vi "CaseStructure Create Case Calls.vi"(9 "Output variables assignements":string[](array[string]), 10 "Frames code[]":string[](array[string]), 11 "FrameNames in":string[](array[string])) -> (2 "Switch Cases C calls all as string":string, 3 "Switch Cases C string array":string[](array[string]))   [LabVIEW 2014]
doc: "Creates case calls for switch(){case \"someName\": break;} and returns them as array."
panel:
  # "Each case \"\" has output variables, so there is way how to get some value from them."
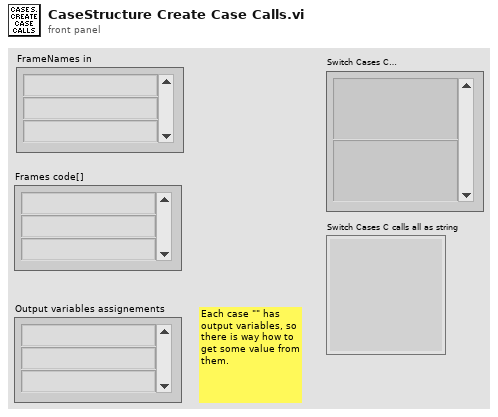
[diagram p1: front panel]
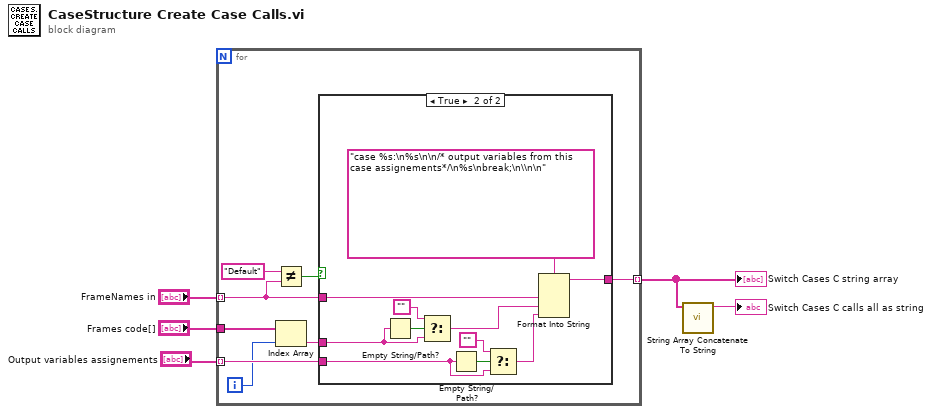
[diagram p0: block diagram]
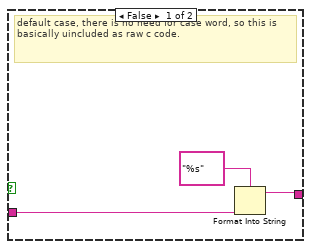
[diagram p2: hidden frame]
diagram:
  n1 = for {
    tunnel: "FrameNames in" -> [w11] mode=indexing
    tunnel: "Frames code[]" -> [w8]
    tunnel: [w12] -> w3 mode=indexing
    tunnel: "Output variables assignements" -> [w13] mode=indexing
    i -> [w7]
    n2 = Not Equal?(x="Default", y=w11) -> (x != y?=w9:bool)
    n3 = Index Array(array=w8, index=w7) -> (element=w6:string)
    n4 = case shown="True" w9 {
      tunnel: w6 -> [_ w21]
      tunnel: w13 -> [_ w17]
      tunnel: [w15 w24] -> w12
      tunnel: w11 -> [w14 w23]
      frame False {
        # "default case, there is no need for case word, so this is basically uincluded as raw c code."
        n5 = Format Into String(format string="%s", w14) -> (resulting string=w15:string)  [unwired: 2 in, 1 out]
      }
      frame True {
        n6 = Empty String/Path?(string/path=w21) -> (empty?=w27:bool)
        n7 = Select(t="", s=w27, f=w21) -> (s? t:f=w25:string)
        n8 = Empty String/Path?(string/path=w17) -> (empty?=w19:bool)
        n9 = Select(t="", s=w19, f=w17) -> (s? t:f=w18:string)
        n10 = Format Into String(format string="case %s:\n%s\n\n/* output variables from this case assignements*/\n%s\nbreak;\n\\n\n", w23, w25, w18) -> (resulting string=w24:string)  [unwired: 2 in, 1 out]
      }
    }
  }
  "Switch Cases C string array" <- w3
  n11 = call "String Array Concatenate To String.vi"("Array String In"=w3) -> ("String"=→"Switch Cases C calls all as string":string)  [unwired: 10 in]
